vi "Motor Control.vi"() -> ()   [LabVIEW 2012]
doc: "<B>Motor Control.vi</B> demonstrates simplistic control of a motor using PWM."
uses:
  StateMachineEnum.ctl
  <vilib>/Rock Robotics/SystemInterfaces/DIO/FPGA_DIOPWMChannel.ctl
  <vilib>/Rock Robotics/SystemInterfaces/Typedef/FPGA_TypedefDigitalModule.ctl
  <vilib>/Rock Robotics/SystemInterfaces/DIO/FPGA_DIOChannel.ctl
  <vilib>/Rock Robotics/WPI/Encoder/WPI_EncoderType.ctl
  <vilib>/Rock Robotics/WPI/MotorControl/WPI_MotorControlOpen Talon.vi
  <vilib>/Rock Robotics/WPI/Counter/WPI_CounterDigitalInputToDigitalSource.vi
  <vilib>/addons/control/pid/pid.llb/PID (DBL).vi
  <vilib>/addons/control/pid/NI_PID_pid.lvlib
panel:
  out "Waveform Chart":cluster{"output":dbl, "Desired RPM":dbl}(graph)
  in  "Manual Contol?":bool
  in  "Motor Manual":dbl(slide) step=0.1 scale=-1.0..1.0
  in  "Desired RPM":dbl step=1.0
  out "Current RPM":dbl
  in  "PID L":T1={"proportional gain (Kc)"=0.0008, "integral time (Ti, min)"=0.01, "derivative time (Td, min)"=0.0} {"derivative time (Td, min)" step=0.01 scale=0.0..0.5; "integral time (Ti, min)" step=0.01 scale=0.0..0.5; "proportional gain (Kc)" step=0.0001 scale=0.0..0.5}
  in  "Output L":cluster{"output high":dbl, "output low":dbl}={"output high"=1.0, "output low"=0.0} {"output low" step=0.1 scale=0.0..1.0; "output high" step=0.1 scale=0.0..1.0}
  in  "Stop":bool=TRUE
  out "Victor LED":bool
  # "Wiring Diagram for Digital Sidecar connected to an NI 9403"
  # "Set these inputs before running."
  # "This can be set while running."
  # "Digital Sidecar"
  # "Power\nTerminals"
  # "Motor\nTerminals"
  # "PWM cable"
  # "This shows wiring for a Victor speed controller.  The wiring is similar for a Luminary Micro Jaguar speed controller.  For a Jaguar, you must also select the appropriate instance of the Motor Open VI on the diagram."
  # "V-"
  # "M-"
  # "V+"
  # "M+"
  # "B"
  # "Innovation First"
  # "VICTOR 884"
  # "B"
  # "C"
  # "PWR"
  # "SIG"
  # "(-)"
  # "+V"
  # "10"
  # "9"
  # "8"
  # "7"
  # "6"
  # "5"
  # "4"
  # "3"
  # "2"
  # "1"
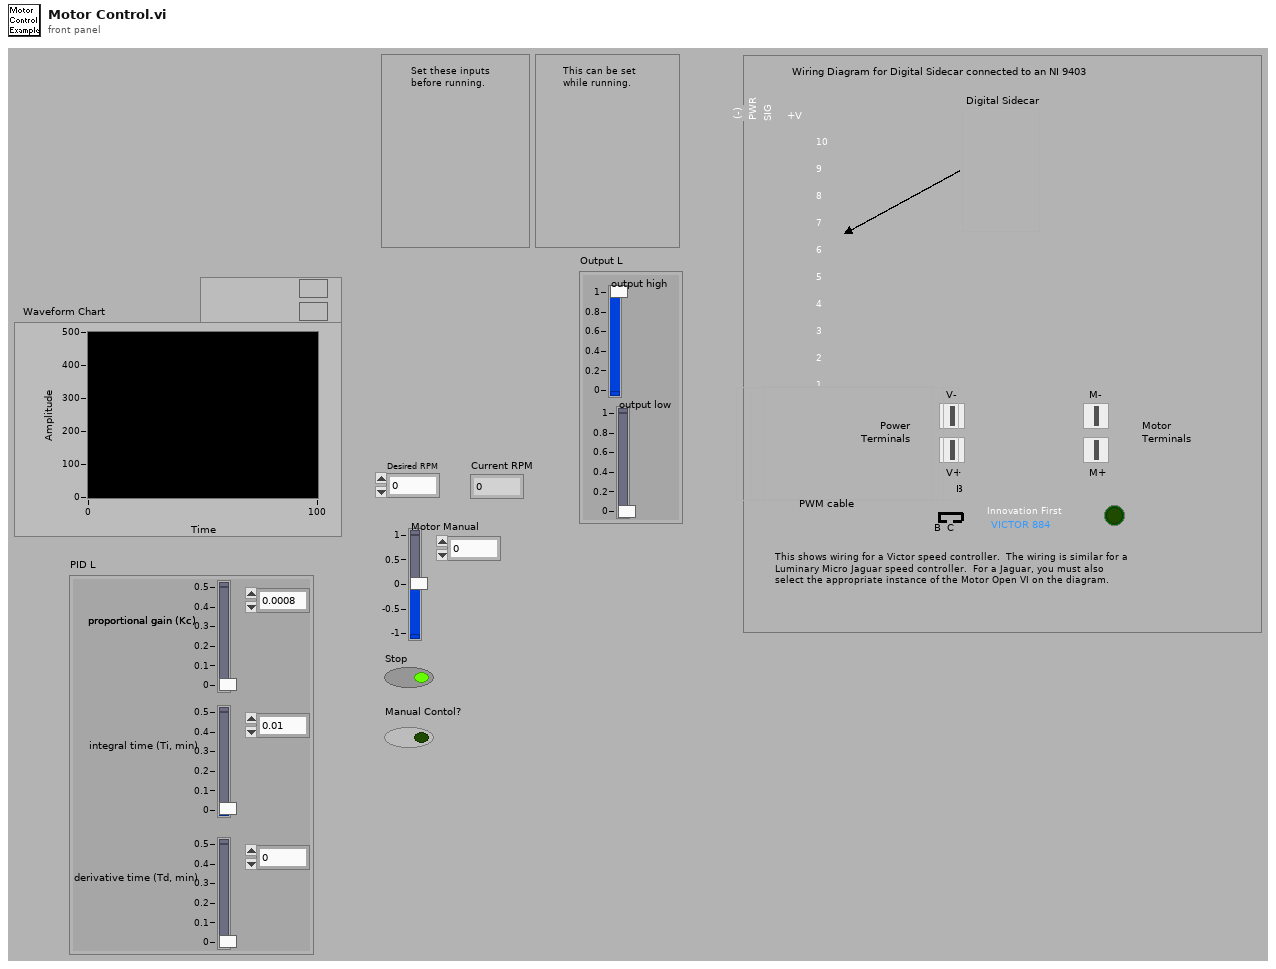
[diagram p1: front panel]
types:
  T1 = cluster{"proportional gain (Kc)":dbl, "integral time (Ti, min)":dbl, "derivative time (Td, min)":dbl}
  T2 = typedef "StateMachineEnum.ctl" = enum16{"Init", "Idle", "Start", "Do", "Stop"}
  T3 = typedef "WPI_EncoderType.ctl" = enum16{"1x", "2x", "4x"}
  T4 = typedef "FPGA_DIOChannel.ctl" = enum8{"DIO 1", "DIO 2", "DIO 3", "DIO 4", "DIO 5", "DIO 6", "DIO 7", "DIO 8", "DIO 9", "DIO 10", "DIO 11", "DIO 12", "DIO 13", "DIO 14", "Invalid"}
  T5 = typedef "FPGA_TypedefDigitalModule.ctl" = enum16{"Digital Module 1", "Digital Module 2"}
  T6 = typedef "FPGA_DIOPWMChannel.ctl" = enum8{"PWM 1", "PWM 2", "PWM 3", "PWM 4", "PWM 5", "PWM 6", "PWM 7", "PWM 8", "PWM 9", "PWM 10", "Invalid"}
  T7 = typedef "WPI_DigitalInputDevRef.ctl" = cluster{"DevStatus":errorcluster, "DIO Channel":T4, "Digital Module":T5}
  T8 = typedef "FPGA_CounterEncoderSourceConvertionLVSourceType.ctl" = cluster{"DevStatus":errorcluster, "AnalogTriggerMode?":bool, "DigitalMode":cluster{"Digital Module":T5, "DIO Channel":T9}, "AnalogTriggerMode":cluster{"AnalogTriggerIndex":T10, "OutputType":T11}}
  T9 = typedef "FPGA_DIODigitalSourceChannel.ctl" = enum8{"DIO 1", "DIO 2", "DIO 3", "DIO 4", "DIO 5", "DIO 6", "DIO 7", "DIO 8", "DIO 9", "DIO 10", "DIO 11", "DIO 12", "DIO 13", "DIO 14", "Disabled"}
  T10 = typedef "FPGA_AnalogTriggerIndex.ctl" = enum8{"Trig 0", "Trig 1", "Trig 2", "Trig 3", "Trig 4", "Trig 5", "Trig 6", "Trig 7", "Invalid"}
  T11 = typedef "FPGA_AnalogTriggerOutType.ctl" = enum16{"InWindow", "TriggerState", "Rising", "Falling"}
  T12 = typedef "WPI_EncoderDevRef.ctl" = cluster{"DevStatus":errorcluster, "EncoderIndex":T13, "CounterIndex":T14, "DistancePerCount":dbl, "Decoding Type":T3}
  T13 = typedef "FPGA_EncoderIdx.ctl" = enum8{"Enc 0", "Enc 1", "Enc 2", "Enc 3", "Invalid"}
  T14 = typedef "FPGA_CounterCtrSystemIndex.ctl" = enum8{"Ctr 0", "Ctr 1", "Ctr 2", "Ctr 3", "Ctr 4", "Ctr 5", "Ctr 6", "Ctr 7", "Invalid"}
  T15 = typedef "WPI_MotorControlDeviceRef.ctl" = cluster{"DeviceStatus":errorcluster, "Type":enum16{"PWM", "CAN"}, "PWM":cluster{"Digital Module":T5, "PWM Channel":T6, "DeadBand":T16}, "CAN":cluster{"Device Number":u8, "Control Mode":T17, "Semaphore":T18, "Max Vout":dbl}, "Invert":bool, "TransformRef":T19, "InvTransformRef":T19}
  T16 = typedef "WPI_PWMDeadband.ctl" = cluster{"Name":string, "maxPositivePwm":i32, "minPositivePwm":i32, "centerPwm":i32, "maxNegativePwm":i32, "minNegativePwm":i32, "angularRange":u16}
  T17 = typedef "WPI_CANJaguar_ControlMode.ctl" = enum8{"Percent VBus", "Current", "Speed", "Position", "Voltage"}
  T18 = typedef "Semaphore RefNum" = refnum<k1>
  T19 = typedef "WPI_PWMTransform_ConPane.ctl" = refnum<vi>
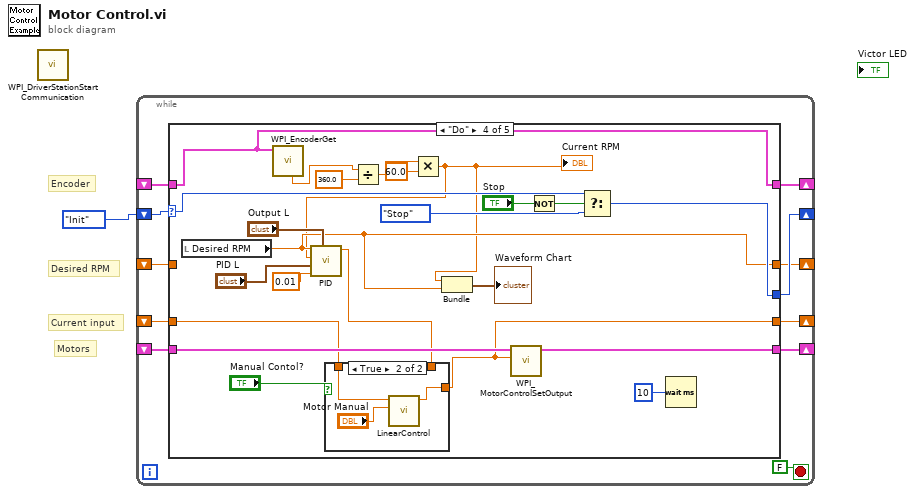
[diagram p0: block diagram]
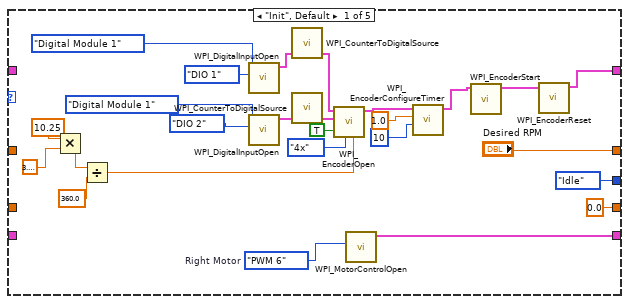
[diagram p2: hidden frame]
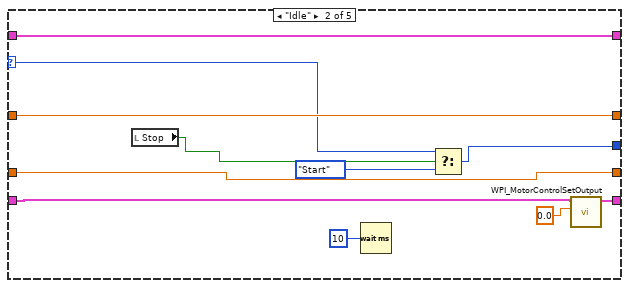
[diagram p3: hidden frame]
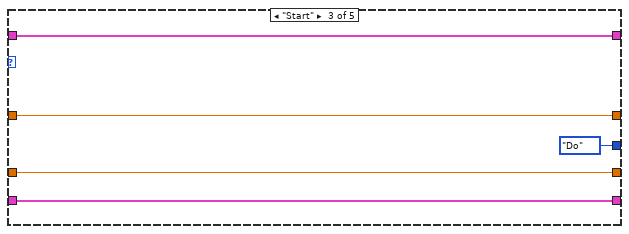
[diagram p4: hidden frame]
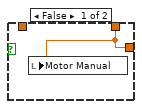
[diagram p5: hidden frame]
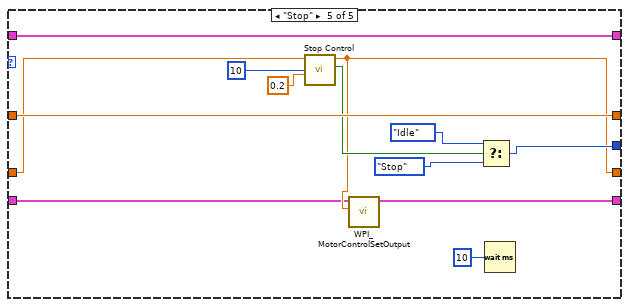
[diagram p6: hidden frame]
diagram:
  # "Current input"
  # "Desired RPM"
  # "Motors"
  # "Encoder"
  n1 = call <vilib>:"WPI_DriverStationStart Communication.vi"() -> ()  [unwired: 1 in, 11 out]
  n2 = while {
    shift-right: [w8] -> _
    shift-left: StateMachineEnum."Init" -> [w11]
    shift-right: [w10] -> _
    shift-left: _ -> [w9]
    shift-right: [w7] -> _
    shift-left: _ -> [w6]
    shift-right: [w5] -> _
    shift-left: _ -> [w4]
    shift-right: [w3] -> _
    shift-left: _ -> [w2]
    stop <- FALSE stop-if-true
    n3 = case shown="\"Do\"" w11 {
      selector: w11 -> [_ w40 _ w77 _]
      tunnel: [w36 w49 w53 w74 w94] -> w10
      tunnel: w9 -> [_ w44 w53 w61 w82]
      tunnel: [StateMachineEnum."Idle" w46 StateMachineEnum."Do" w75 w84] -> w8
      tunnel: [w13 w48 w52 w64 w92] -> w7
      tunnel: w6 -> [_ w48 w52 w64 w92]
      tunnel: ["Desired RPM" w47 w51 w58 w93] -> w5
      tunnel: w4 -> [_ w47 w51 _ w93]
      tunnel: [0.0 ("New Motor Input") w45 w50 w60 w83] -> w3
      tunnel: w2 -> [_ w45 w50 w59 w90]
      frame "Init", Default {
        w37 = FPGA_DIOPWMChannel."PWM 6"  # Right Motor
        n4 = Multiply(x=10.25, y=3.141592653589793) -> (x*y=w21:dbl)
        n5 = Divide(x=w21, y=360.0) -> (x/y=w19:dbl)
        n6 = call <vilib>:"WPI_DigitalInputOpen.vi"("DIO Channel"=FPGA_DIOChannel."DIO 1", "Digital Module (Module 1)"=FPGA_TypedefDigitalModule."Digital Module 1") -> ("DigitalInputDevRef"=w33:T7)  [unwired: 1 in, 8 out]
        n7 = call <vilib>:"WPI_DigitalInputOpen.vi"("DIO Channel"=FPGA_DIOChannel."DIO 2", "Digital Module (Module 1)"=FPGA_TypedefDigitalModule."Digital Module 1") -> ("DigitalInputDevRef"=w34:T7)  [unwired: 1 in, 8 out]
        n8 = call-poly <vilib>:"WPI_CounterToDigitalSource.vi"("DigitalInputDevRef"=w33) -> ("Digital Source"=w32:T8)  [unwired: 6 out]
        n9 = call-poly <vilib>:"WPI_CounterToDigitalSource.vi"("DigitalInputDevRef"=w34) -> ("Digital Source"=w35:T8)  [unwired: 6 out]
        n10 = call <vilib>:"WPI_EncoderOpen.vi"("DistancePerCount"=w19, "Decoding Type"=WPI_EncoderType."4x", "Invert Direction (False)"=TRUE, "BSource"=w35, "ASource"=w32) -> ("EncoderDevRef"=w29:T12)  [unwired: 3 in, 3 out]
        n11 = call-poly <vilib>:"WPI_MotorControlOpen.vi"("PWM Channel"=w37) -> ("MotorControlDeviceRef"=w36:T15)  [unwired: 9 in, 1 out]
        n12 = call <vilib>:"WPI_EncoderConfigureTimer.vi"("Number Samples to Average"=u8 10, "Minimum Rate"=1.0, "EncoderDevRef"=w29) -> ("EncoderDevRef"=w15:T12)  [unwired: 1 in, 7 out]
        n13 = call <vilib>:"WPI_EncoderStart.vi"("EncoderDevRef"=w15) -> ("EncoderDevRef"=w14:T12)  [unwired: 9 in, 1 out]
        n14 = call <vilib>:"WPI_EncoderReset.vi"("EncoderDevRef"=w14) -> ("EncoderDevRef"=w13:T12)  [unwired: 9 in, 1 out]
      }
      frame "Idle" {
        n15 = local read "Stop"() -> (w42:bool)
        n16 = Wait (ms)(milliseconds to wait=u32 10) -> ()  [unwired: 1 out]
        n17 = Select(t=w40, s=w42, f=StateMachineEnum."Start") -> (s? t:f=w46:T2)
        n18 = call <vilib>:"WPI_MotorControlSetOutput.vi"("Output"=0.0, "MotorControlDevRef"=w44) -> ("MotorControlDevRef"=w49:T15)  [unwired: 7 in, 2 out]
      }
      frame "Start" {
      }
      frame "Do" {
        n19 = local read "Desired RPM"() -> (w58:dbl)
        n20 = call <vilib>:"WPI_EncoderGet.vi"("EncoderDevRef"=w64) -> ("Rate"=w71:dbl)  [unwired: 5 in, 5 out]
        n21 = Divide(x=w71, y=360.0) -> (x/y=w69:dbl)
        n22 = Multiply(x=w69, y=60.0) -> (x*y=w55:dbl)
        "Current RPM" <- w55
        n23 = call-poly <vilib>:"PID.vi"("output range"="Output L", "dt (s)"=0.01, "PID gains"="PID L", "process variable"=w55, "setpoint"=w58) -> ("output"=w56:dbl)  [unwired: 5 in, 1 out]
        n24 = case shown="True" "Manual Contol?" {
          tunnel: [w78 w79] -> w60
          tunnel: w56 -> [w78 _]
          tunnel: w59 -> [_ w80]
          frame False {
            n25 = local write "Motor Manual"(w78) -> ()
          }
          frame True {
            n26 = call "LinearControl.vi"("Setpoint"="Motor Manual", "Motor Value"=w80) -> ("New Motor Value"=w79:dbl)  [unwired: 8 in, 1 out]
          }
        }
        n27 = Bundle(w55, "Desired RPM"=w58) -> (→"Waveform Chart":cluster{dbl, "Desired RPM":dbl})  [unwired: 1 in]
        n28 = call <vilib>:"WPI_MotorControlSetOutput.vi"("Output"=w60, "MotorControlDevRef"=w61) -> ("MotorControlDevRef"=w74:T15)  [unwired: 7 in, 2 out]
        n29 = Not(x="Stop") -> (.not. x?=w63:bool)
        n30 = Select(t=w77, s=w63, f=StateMachineEnum."Stop") -> (s? t:f=w75:T2)
        n31 = Wait (ms)(milliseconds to wait=u32 10) -> ()  [unwired: 1 out]
      }
      frame "Stop" {
        n32 = call "Stop Control.vi"("Rate (unit/s)"=0.2, "Loop Time (ms)"=u32 10, "Recieved Motor Input"=w90) -> ("Done Stopping"=w87:bool, "New Motor Input"=w83:dbl)  [unwired: 7 in]
        n33 = call <vilib>:"WPI_MotorControlSetOutput.vi"("Output"=w83, "MotorControlDevRef"=w82) -> ("MotorControlDevRef"=w94:T15)  [unwired: 7 in, 2 out]
        n34 = Select(t=StateMachineEnum."Idle" ("f"), s=w87, f=StateMachineEnum."Stop") -> (s? t:f=w84:T2)
        n35 = Wait (ms)(milliseconds to wait=u32 10) -> ()  [unwired: 1 out]
      }
    }
  }
